vi "Get Database Information v1_0_0.vi"(6 "Use Fast quarry":bool=TRUE, 7 "Table name":string="devvehlist", 8 "error in":errorcluster, 9 "table index":i32, 10 "show all\nTables?":bool, 11 "connection information":path=path "C:/Documents and Settings/Owner/My Documents/AM/Projects/HRA/HRA_Suspension_Test_System/HRA.udl") -> (0 "error out":errorcluster, 2 "Data Array":string[][](array[string])=[["1", "2", "3", "4", "5", "6", "7", "8", "9", "10", "11", "12", "13", "14", "15", "16", "17", "18", "19", "20"], ["Select one", "Other", "KA", "KB", "KC", "KD", "KE", "KG", "KJ", "KK", "KL", "KM", "KN", "KP", "KQ", "KS", "KT", "KV", "KX", "KY"], ["Select one", "Other", "Convertible", "Coupe", "Hatchback", "Sedan", "SUV", "Truck", "Van", "Wagon", "", "", "", "", "", "", "", "", "", ""], ["Select one", "Other", "1", "2", "3", "4", "5", "6", "7", "8", "9", "", "", "", "", "", "", "", "", ""], ["Select one", "Other", "N", "Y", "", "", "", "", "", "", "", "", "", "", "", "", "", "", "", ""], ["Select one", "Other", "FF", "FR", "MR", "RR", "F 4WD", "R 4WD", "", "", "", "", "", "", "", "", "", "", "", ""], ["Select one", "Other", "Longitudinal", "Transverse", "", "", "", "", "", "", "", "", "", "", "", "", "", "", "", ""], ["Select one", "Other", "I3", "I4", "I5", "I6", "I8", "V4", "V5", "V6", "V8", "V10", "V12", "Flat 4", "Flat 6", "Flat 12", "", "", "", ""], ["Select one", "Other", "3MT", "4MT", "5MT", "6MT", "7MT", "3AT", "4AT", "5AT", "6AT", "7AT", "", "", "", "", "", "", "", ""], ["Select one", "Other", "LH", "RH", "Center", "", "", "", "", "", "", "", "", "", "", "", "", "", "", ""], ["Select one", "Other", "BFGoodrich", "Bridgestone", "Continental", "Cooper", "Dunlop", "Firestone", "General", "Goodyear", "Kumho", "Michelin", "Pirelli", "Sumitoma", "Uniroyal", "Yokahama", "", "", "", ""], ["Select one", "Other", "H", "S", "T", "U", "V", "W", "Y", "ZR", "", "", "", "", "", "", "", "", "", ""], ["Select one", "Other", "J", "JJ", "", "", "", "", "", "", "", "", "", "", "", "", "", "", "", ""], ["Select one", "Other", "BFGoodrich", "Bridgestone", "Continental", "Cooper", "Dunlop", "Firestone", "General", "Goodyear", "Kumho", "Michelin", "Pirelli", "Sumitoma", "Uniroyal", "Yokahama", "", "", "", ""], ["Select one", "Other", "H", "S", "T", "U", "V", "W", "Y", "ZR", "", "", "", "", "", "", "", "", "", ""], ["Select one", "Other", "J", "JJ", "", "", "", "", "", "", "", "", "", "", "", "", "", "", "", ""], ["Select one", "Other", "MacPherson Strut", "SLA", "Trailing Arm", "Four Link", "", "", "", "", "", "", "", "", "", "", "", "", "", ""], ["Select one", "Other", "MacPherson Strut", "SLA", "Trailing Arm", "Semi-trailing Arm", "Swing Axle", "Hotchkiss", "Four Link (solid axle)", "de Dion", "", "", "", "", "", "", "", "", "", ""], ["Select one", "Other", "D1", "PO", "P1", "T-Step", "", "", "", "", "", "", "", "", "", "", "", "", "", ""], ["Select one", "Other", "Bumpstop", "Compliances", "Damper", "Kinematics", "Spring Rates", "Stabilizer Bar", "Tire", "Validation", "", "", "", "", "", "", "", "", "", ""], ["Select one", "Other", "S9VA", "SEPA", "", "", "", "", "", "", "", "", "", "", "", "", "", "", "", ""], ["Other", "Large Vehicle Picture", "Large Vehicle Picture", "Large Vehicle Picture", "Large Vehicle Picture", "Large Vehicle Picture", "Large Vehicle Picture", "Large Vehicle Picture", "Large Vehicle Picture", "Large Vehicle Picture", "Large Vehicle Picture", "Large Vehicle Picture", "Large Vehicle Picture", "Large Vehicle Picture", "Large Vehicle Picture", "Large Vehicle Picture", "", "", "", ""]], 3 "Database Information":string[][](table)=[["devvehlist", "ID", "Long (I32)", "-1"], ["", "Market", "String", "-1"], ["", "Body_Style", "String", "-1"], ["", "Doors", "String", "-1"], ["", "Sunroof", "String", "-1"], ["", "Powertrain_L_O", "String", "-1"], ["", "Engine_L_O", "String", "-1"], ["", "Engine_Type", "String", "-1"], ["", "Transmission", "String", "-1"], ["", "Str_Position", "String", "-1"], ["", "F_Tire_Make", "String", "-1"], ["", "F_Tire_SR", "String", "-1"], ["", "F_Whl_Shape", "String", "-1"], ["", "R_Tire_Make", "String", "-1"], ["", "R_Tire_SR", "String", "-1"], ["", "R_Whl_Shape", "String", "-1"], ["", "F_Sus_Type", "String", "-1"], ["", "R_Sus_Type", "String", "-1"], ["", "Project_Timing", "String", "-1"], ["", "Tuning_Item", "String", "-1"], ["", "Frame_Code", "String", "-1"], ["", "Vehicle_Picture", "String", "-1"]])   [LabVIEW 2009]
doc: "Get Database Information v1_0_0.vi\n\nThis example returns information contained in a database. The information consists of the table names, column names, data types, and data sizes.\n\n\ncreated 2002\nby J. Daren Suntych\nNational Analytics\n970-397-0764"
uses:
  <vilib>/addons/database/Connection.llb/DB Tools Open Connec (Path).vi
  <vilib>/addons/database/NI_Database_API.lvlib
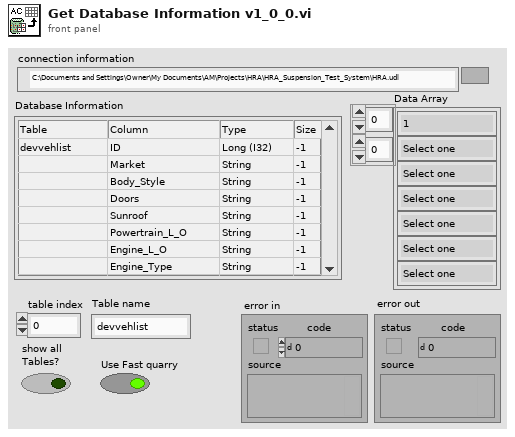
[diagram p1: front panel]
types:
  T1 = typedef "NI_Database_API.lvlib/Conn ObjectReference.ctl" = refnum<k1>
  T2 = typedef "NI_Database_API.lvlib/DB Tools DataTypes.ctl" = enum16{"String", "Long (I32)", "Single (SGL)", "Double (DBL)", "Date/Time", "Binary"}
  T3 = cluster{"name":string, "database data type":T2, "defined size":i32}[]
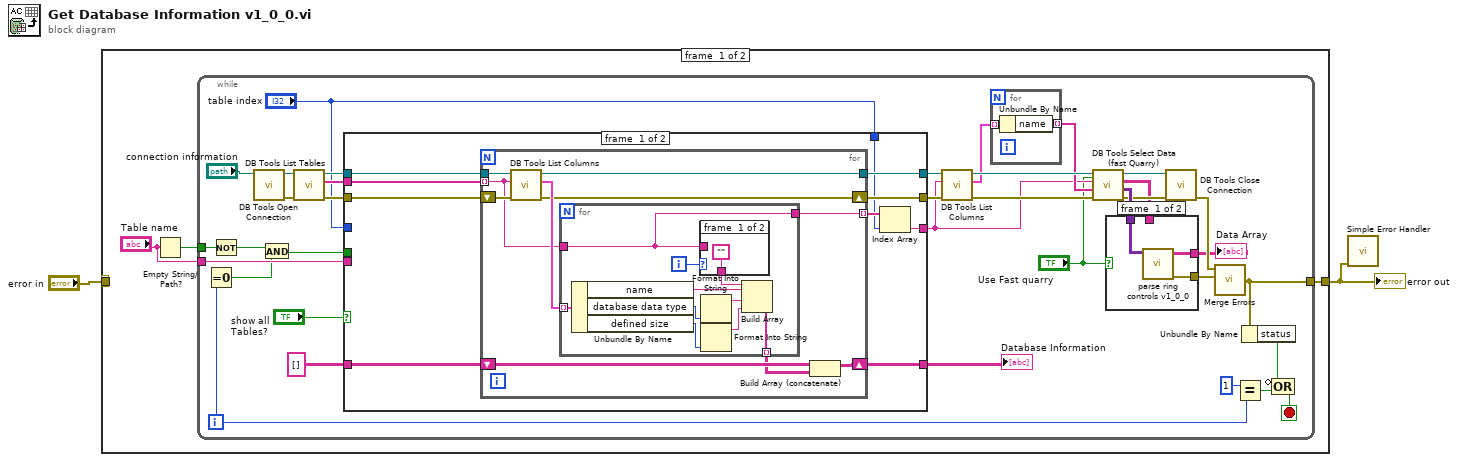
[diagram p0: block diagram]
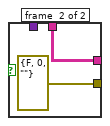
[diagram p2: hidden frame]
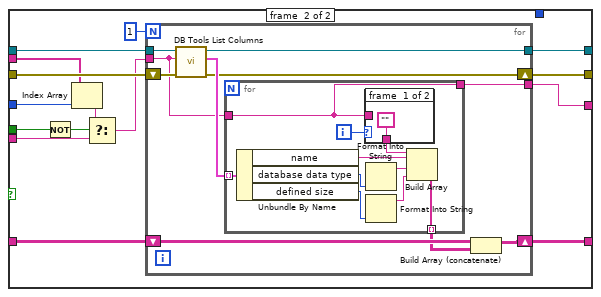
[diagram p4: hidden frame]
diagram:
  n1 = case shown="No Error" "error in" {
    tunnel: [w5 w118] -> w1
    tunnel: "error in" -> [_ w118]
    frame #0 {
      n2 = Empty String/Path?(string/path="Table name") -> (empty?=w3:bool)
      n3 = while {
        tunnel: [w17] -> w5
        tunnel: "Table name" -> [w22]
        tunnel: w3 -> [w20]
        i -> [w16]
        stop <- w12 stop-if-true
        n4 = Equal To 0?(x=w16) -> (x = 0?=w21:bool)
        n5 = Not(x=w20) -> (.not. x?=w18:bool)
        n6 = call-poly <vilib>:"DB Tools Open Connection.vi"("connection information"="connection information") -> ("error out"=w41:errorcluster, "connection reference"=w40:T1)  [unwired: 7 in]
        n7 = And(x=w18, y=w21) -> (x .and. y?=w19:bool)
        n8 = call <vilib>:"DB Tools List Tables.vi"("error in (no error)"=w41, "connection reference"=w40) -> ("error out"=w38:errorcluster, "tables"=w37:string[], "connection reference out"=w39:T1)  [unwired: 3 in]
        n9 = case shown="False" "show all\nTables?" {
          tunnel: w39 -> [w56 w93]
          tunnel: w38 -> [w55 w92]
          tunnel: w37 -> [w54 w86]
          tunnel: [w53 w91] -> w36
          tunnel: string[][] [] -> [w52 w90]
          tunnel: [w47 w89] -> w10
          tunnel: [w51 w88] -> w30
          tunnel: [w50 w87] -> w27
          tunnel: "table index" -> [_ w85]
          tunnel: w19 -> [_ w81]
          tunnel: w22 -> [_ w80]
          tunnel: "table index" -> [w48 _]
          frame #0 {
            n10 = for {
              tunnel: w56 -> [w65]
              shift-right: [w59] -> w50
              shift-left: w55 -> [w66]
              tunnel: w54 -> [w57] mode=indexing
              shift-right: [w64] -> w53
              shift-left: w52 -> [w63]
              tunnel: [w61] -> w51
              tunnel: [w58] -> w49 mode=indexing
              n11 = call <vilib>:"DB Tools List Columns.vi"("error in (no error)"=w66, "table"=w57, "connection reference"=w65) -> ("error out"=w59:errorcluster, "column information"=w60:T3, "connection reference out"=w61:T1)  [unwired: 1 in, 1 out]
              n12 = for {
                tunnel: w57 -> [w67]
                tunnel: w60 -> [w73] mode=indexing
                tunnel: [w75] -> w62 mode=indexing
                tunnel: [w67] -> w58
                i -> [w76]
                n13 = Unbundle By Name(w73) -> ("name"=w68:string, "database data type"=w72:T2, "defined size"=w70:i32)
                n14 = case shown="0" w76 {
                  tunnel: w67 -> [_ w78]
                  tunnel: ["" w78] -> w74
                  frame #0 {
                  }
                  frame #1 {
                  }
                }
                n15 = Format Into String(w72) -> (resulting string=w71:string)  [unwired: 3 in, 1 out]
                n16 = Format Into String(w70) -> (resulting string=w69:string)  [unwired: 3 in, 1 out]
                n17 = Build Array(w74, w68, w71, w69) -> (w75:string[])
              }
              n18 = Build Array (concatenate)(w63, w62) -> (w64:string[][])
            }
            n19 = Index Array(array=w49, index=w48) -> (element=w47:string)
          }
          frame #1 {
            n20 = Not(x=w81) -> (.not. x?=w79:bool)
            n21 = Index Array(array=w86, index=w85) -> (element=w82:string)
            n22 = Select(t=w82, s=w79, f=w80) -> (s? t:f=w83:string)
            n23 = for {
              N: 1 -> [_]
              tunnel: w93 -> [w102]
              shift-right: [w96] -> w87
              shift-left: w92 -> [w103]
              tunnel: w83 -> [w94]
              shift-right: [w101] -> w91
              shift-left: w90 -> [w100]
              tunnel: [w98] -> w88
              tunnel: [w95] -> w89
              n24 = call <vilib>:"DB Tools List Columns.vi"("error in (no error)"=w103, "table"=w94, "connection reference"=w102) -> ("error out"=w96:errorcluster, "column information"=w97:T3, "connection reference out"=w98:T1)  [unwired: 1 in, 1 out]
              n25 = for {
                tunnel: w94 -> [w104]
                tunnel: w97 -> [w110] mode=indexing
                tunnel: [w112] -> w99 mode=indexing
                tunnel: [w104] -> w95
                i -> [w113]
                n26 = Unbundle By Name(w110) -> ("name"=w106:string, "database data type"=w109:T2, "defined size"=w105:i32)
                n27 = case shown="Default" w113 {
                  tunnel: w104 -> [_ w115]
                  tunnel: ["" w115] -> w111
                  frame #0 {
                  }
                  frame #1 {
                  }
                }
                n28 = Format Into String(w109) -> (resulting string=w108:string)  [unwired: 3 in, 1 out]
                n29 = Format Into String(w105) -> (resulting string=w107:string)  [unwired: 3 in, 1 out]
                n30 = Build Array(w111, w106, w108, w107) -> (w112:string[])
              }
              n31 = Build Array (concatenate)(w100, w99) -> (w101:string[][])
            }
          }
        }
        "Database Information" <- w36
        n32 = call <vilib>:"DB Tools List Columns.vi"("error in (no error)"=w27, "table"=w10, "connection reference"=w30) -> ("error out"=w29:errorcluster, "column information"=w26:T3, "connection reference out"=w31:T1)  [unwired: 1 in, 1 out]
        n33 = for {
          tunnel: w26 -> [w117] mode=indexing
          tunnel: [w116] -> w25 mode=indexing
          n34 = Unbundle By Name(w117) -> ("name"=w116:string)
        }
        n35 = call "DB Tools Select Data (fast Quarry).vi"("Use Fast quarry"="Use Fast quarry", "error in (no error)"=w29, "columns"=w25, "table"=w10, "connection reference"=w31) -> ("error out"=w28:errorcluster, "data"=w32:variant[][], "Data out"=w7:string[][], "connection reference out"=w33:T1)  [unwired: 3 in]
        n36 = case shown="True" "Use Fast quarry" {
          tunnel: w32 -> [w44 _]
          tunnel: [w43 errorcluster {"status"=FALSE, "code"=0, "source"=""} ("error out")] -> w24
          tunnel: [w42 w46] -> w8
          tunnel: w7 -> [_ w46]
          frame #0 {
            n37 = call "parse ring controls v1_0_0.vi"("data"=w44) -> ("error out"=w43:errorcluster, "Array"=w42:string[][])  [unwired: 9 in]
          }
          frame #1 {
          }
        }
        "Data Array" <- w8
        n38 = call <vilib>:"DB Tools Close Connection.vi"("error in (no error)"=w28, "connection reference"=w33) -> ("error out"=w9:errorcluster)  [unwired: 5 in]
        n39 = call <vilib>:"Merge Errors.vi"("error in 2 (no error)"=w24, "error in 1 (no error)"=w9) -> ("error out"=w17:errorcluster)  [unwired: 5 in]
        n40 = Equal?(x=1, y=w16) -> (x = y?=w13:bool)
        n41 = Unbundle By Name(w17) -> ("status"=w15:bool)
        n42 = Compound Arithmetic op=OR(invert w15, w13) -> (w12:bool)
      }
    }
    frame #1 {
    }
  }
  "error out" <- w1
  n43 = call <vilib>:"Simple Error Handler.vi"("error in (no error)"=w1) -> ()  [unwired: 4 in, 5 out]
